vi "Find Connected NI Devices.vi"(8 "error in":errorcluster) -> (0 "error out":errorcluster, 2 "Alias Name(s)":string[](array[string]), 3 "Model(s)":string[](array[string]))   [LabVIEW 2023]
uses:
  <vilib>/nisyscfg/Filter Mode.ctl
  <vilib>/nisyscfg/Close (System).vi
  <vilib>/nisyscfg/nisyscfg.lvlib
  <resource>/objmgr/nisysapi.rc
panel:
  out "size(s)":i32
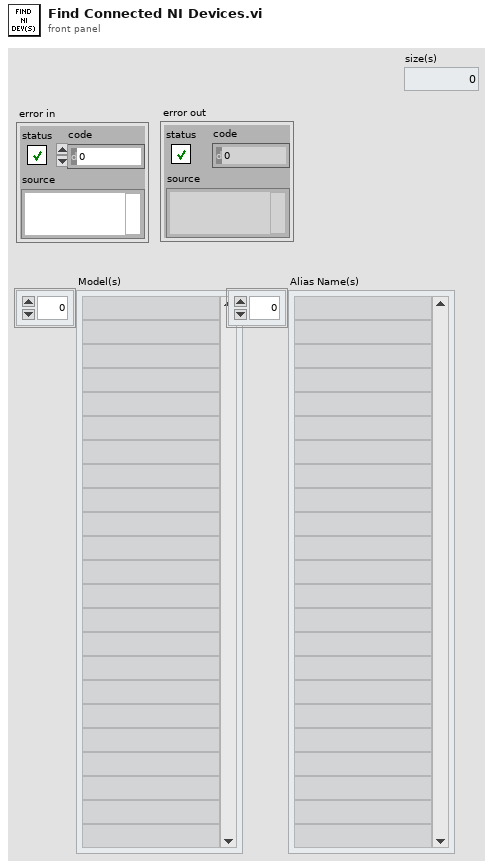
[diagram p1: front panel]
types:
  T1 = typedef "nisyscfg.lvlib/Filter Mode.ctl" = i32
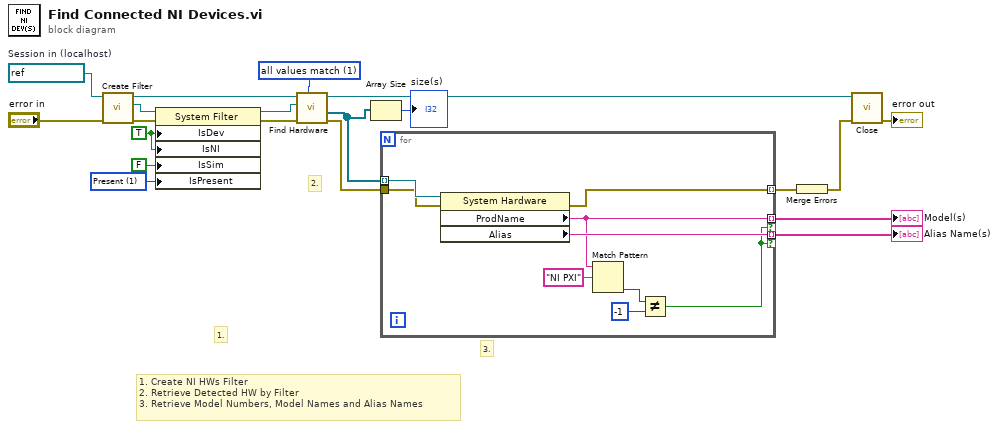
[diagram p0: block diagram]
diagram:
  w1 = 1 items=["Initializing"=-2, "Unknown"=-1, "Not Present"=0, "Present"=1] ("Devices & Chassis:Is Present")
  w20 = refnum<k21> "localhost"  # Session in (localhost)
  w9 = TRUE ("Is Device")
  w3 = T1 1 items=["all values match"=1, "any value matches"=2, "values do not match"=3, "all properties exist"=4] ("Filter Mode (all values match)")
  # "3."
  # "2."
  # "1."
  # "1. Create NI HWs Filter\n2. Retrieve Detected HW by Filter\n3. Retrieve Model Numbers, Model Names and Alias Names"
  n1 = call <vilib>:"Create Filter.vi"("error in (no error)"="error in", "Session in"=w20) -> ("error out"=w12:errorcluster, "Filter out"=w11:refnum<k20>, "Session out"=w8:refnum<k21>)  [unwired: 7 in]
  n2 = property class="System Filter"(reference=w11, error in=w12, "IsDev"=w9, "IsNI"=w9, "IsSim"=FALSE ("Devices & Chassis:Is Simulated"), "IsPresent"=w1) -> (reference out=w2:refnum<k20>, error out=w10:errorcluster)
  n3 = call <vilib>:"Find Hardware.vi"("Filter Mode (all values match)"=w3, "error in (no error)"=w10, "Filter in"=w2, "Session in"=w8) -> ("error out"=w17:errorcluster, "Resources out"=w5:refnum<k20>[], "Session out"=w18:refnum<k21>)  [unwired: 4 in, 1 out]
  n4 = Array Size(array=w5) -> (size(s)=→"size(s)":i32)
  n5 = for {
    tunnel: w5 -> [w27] mode=indexing
    tunnel: w17 -> [w26]
    tunnel: [w29] -> w16 mode=indexing
    tunnel: [w25] -> w14 mode=indexing if=w21
    tunnel: [w28] -> w13 mode=indexing if=w21
    n6 = property class="System Hardware"(reference=w27, error in=w26) -> (error out=w29:errorcluster, "ProdName"=w25:string, "Alias"=w28:string)  [unwired: 1 out]
    n7 = Match Pattern(string=w25, regular expression="NI PXI") -> (offset past match=w23:i32)  [unwired: 1 in, 3 out]
    n8 = Not Equal?(x=w23, y=-1) -> (x != y?=w21:bool)
  }
  "Model(s)" <- w14
  "Alias Name(s)" <- w13
  n9 = Merge Errors(w16) -> (w15:errorcluster)
  n10 = call-poly <vilib>:"Close.vi"("error in (no error)"=w15, "Session in"=w18) -> ("error out"=→"error out":errorcluster)  [unwired: 9 in]
